vi "Physical Constant Selector.vi"(7 "Long / Short ?":bool, 9 "Long Wire Length":dbl, 10 "Short Wire Length":dbl) -> (2 "Wire Length Out":dbl)   [LabVIEW 2015]
panel:
  # "Outputs"
  # "Inputs"
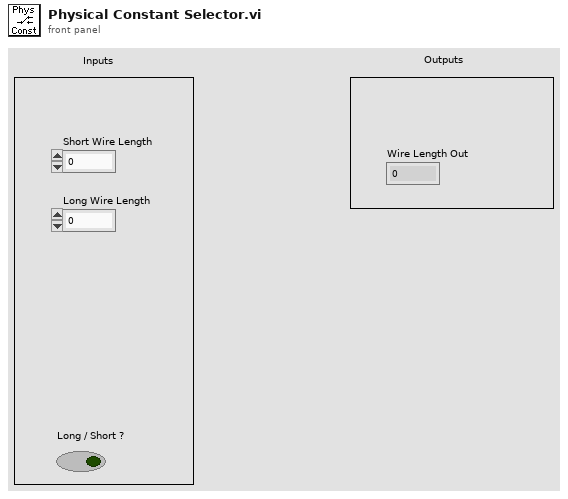
[diagram p1: front panel]
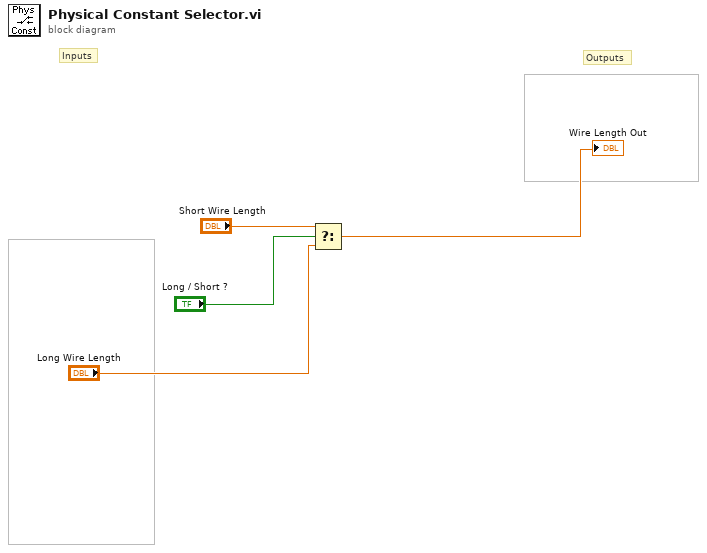
[diagram p0: block diagram]
diagram:
  # "Outputs"
  # "Inputs"
  n1 = Select(t="Short Wire Length", s="Long / Short ?", f="Long Wire Length") -> (s? t:f=→"Wire Length Out":dbl)
